vi "Write Measurement Timeout (ms).vi"(8 "error in (no error)":errorcluster, 10 "Measurement Timeout (ms)":dbl, 11 "ExperimentVariables in":refnum<class "ExperimentVariables.lvclass">) -> (0 "error out":errorcluster, 3 "ExperimentVariables out":refnum<class "ExperimentVariables.lvclass">)   [LabVIEW 2013, in "ExperimentVariables.lvclass"]
uses:
  ExperimentVariables.lvclass
  ExperimentVariables.lvclass/ExperimentVariables.ctl
  Experiment/Globals.vi
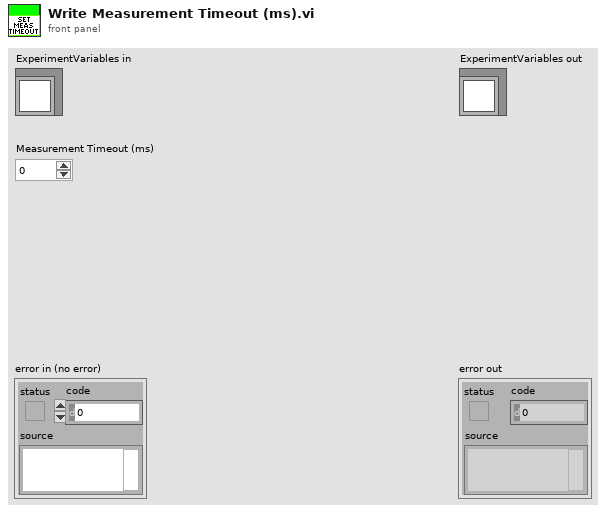
[diagram p1: front panel]
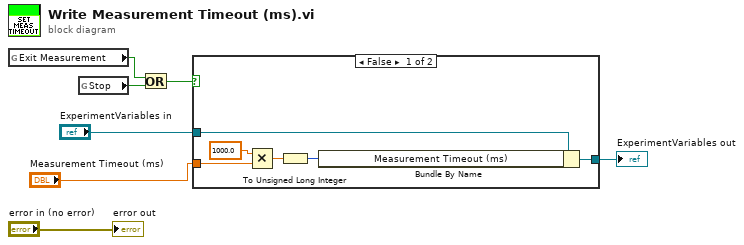
[diagram p0: block diagram]
diagram:
  n1 = global read "Globals.vi" "Exit Measurement"() -> (w4:bool)
  n2 = global read "Globals.vi" "Stop"() -> (w3:bool)
  n3 = Or(x=w4, y=w3) -> (x .or. y?=w2:bool)
  n4 = case shown="False" w2 {
    tunnel: [w12 w14] -> w6
    tunnel: "ExperimentVariables in" -> [w13 w14]
    tunnel: "Measurement Timeout (ms)" -> [w11 _]
    frame False {
      n5 = Multiply(x=1000.0, y=w11) -> (x*y=w9:dbl)
      n6 = To Unsigned Long Integer(number=w9) -> (unsigned 32bit integer=w8:u32)
      n7 = Bundle By Name(cluster=w13, "Measurement Timeout (ms)"=w8) -> (w12:refnum<class "ExperimentVariables.lvclass">)
    }
    frame True {
    }
  }
  "ExperimentVariables out" <- w6
  "error out" <- "error in (no error)"
